vi "test_az_pos.vi"() -> ()   [LabVIEW 2019]
panel:
  out "counts":u64[](graph)
  in  "home":dbl format="%#_13g"
  out "error":dbl[](graph)
  out "graph":dbl[][](graph)
  out "out [deg]":dbl[](array[numeric])
  out "in [deg]":dbl[](array[numeric])
  in  "negate?":bool
  in  "reference":u64=79895940197
  in  "step":u64=4018143232
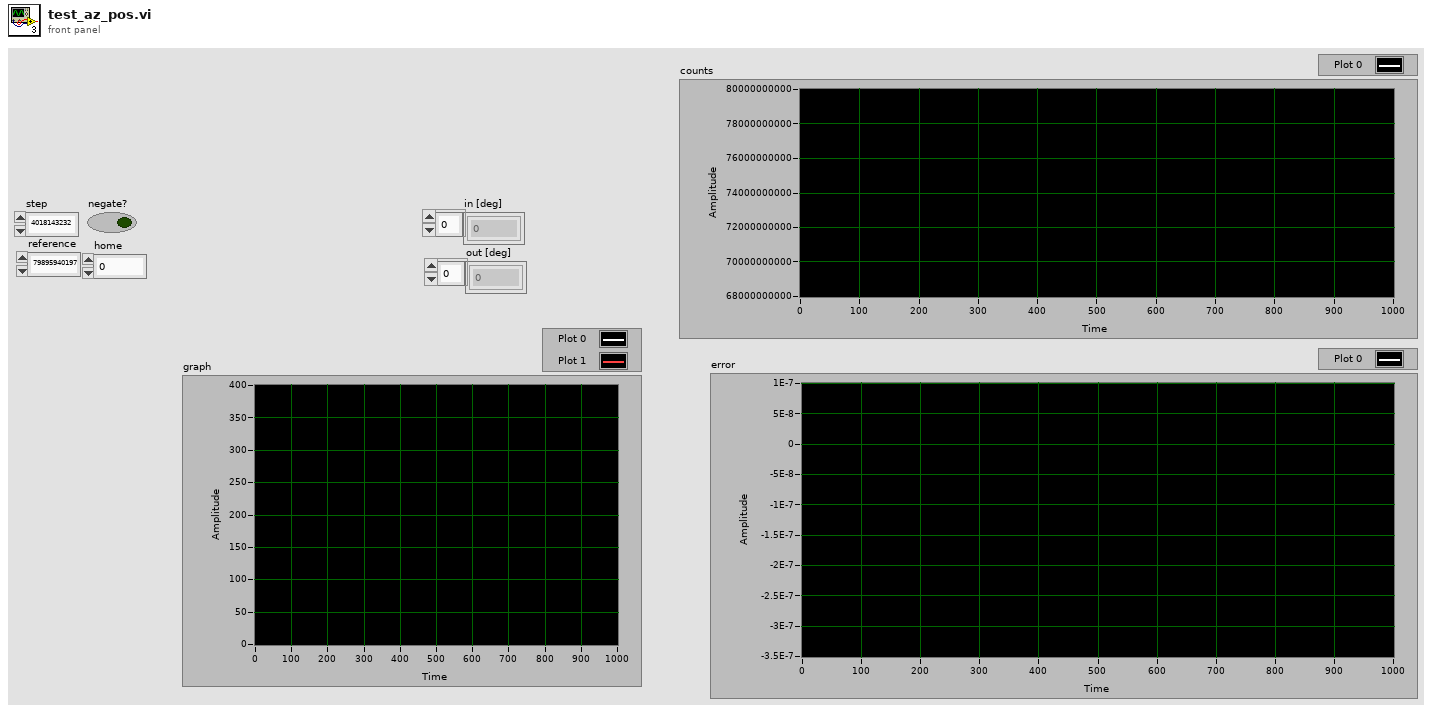
[diagram p1: front panel]
types:
  T1 = cluster{"home":fxp<+/-,32,2>, "counts":u64, "reference":u64, "step":u64, "negate?":bool}
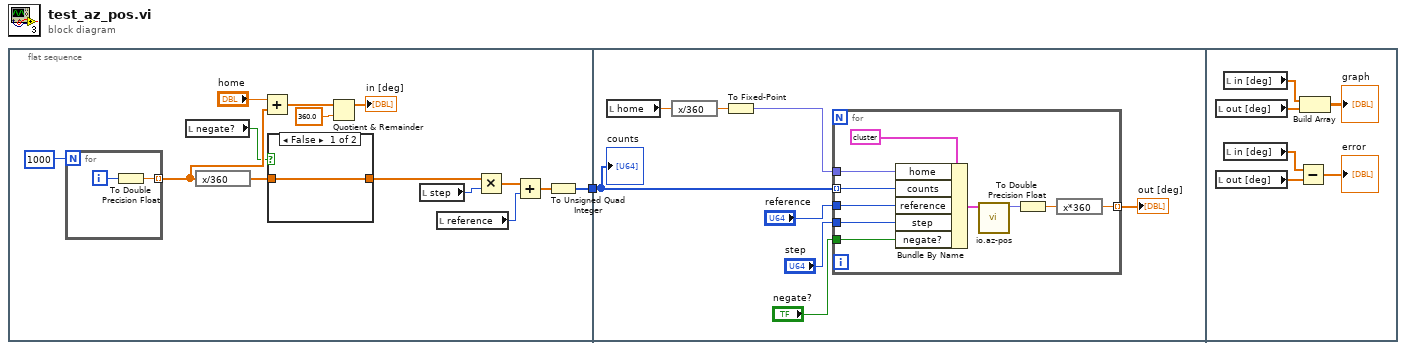
[diagram p0: block diagram]
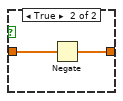
[diagram p2: hidden frame]
diagram:
  n1 = flat-sequence {
    tunnel: [w11] -> w1
    tunnel: w1 -> [w25]
    frame #0 {
      n2 = for {
        N: 1000 -> [_]
        tunnel: [w19] -> w8 mode=indexing
        i -> [w20]
        n3 = To Double Precision Float(number=w20) -> (double precision float=w19:dbl)
      }
      n4 = local read "negate?"() -> (w4:bool)
      n5 = expression code="x/360"(w8) -> (w5:dbl[])
      n6 = Add(x="home", y=w8) -> (x+y=w7:dbl[])
      n7 = case shown="False" w4 {
        tunnel: [w16 w17] -> w3
        tunnel: w5 -> [w16 w18]
        frame False {
        }
        frame True {
          n8 = Negate(x=w18) -> (-x=w17:dbl[])
        }
      }
      n9 = Quotient & Remainder(x=w7, y=360.0) -> (x-y*floor(x/y)=→"in [deg]":dbl[])  [unwired: 1 out]
      n10 = local read "step"() -> (w14:u64)
      n11 = local read "reference"() -> (w13:u64)
      n12 = Multiply(x=w3, y=w14) -> (x*y=w2:dbl[])
      n13 = Add(x=w2, y=w13) -> (x+y=w12:dbl[])
      n14 = To Unsigned Quad Integer(1:w12) -> (0:w11:u64[])
    }
    frame #1 {
      n15 = local read "home"() -> (w23:dbl)
      n16 = expression code="x/360"(w23) -> (w22:dbl)
      n17 = To Fixed-Point(number=w22) -> (fixed-point=w21:fxp<+/-,32,2>)  [unwired: 1 in]
      n18 = for {
        tunnel: [w34] -> w24 mode=indexing
        tunnel: "reference" -> [w33]
        tunnel: "step" -> [w32]
        tunnel: "negate?" -> [w31]
        tunnel: w21 -> [w30]
        tunnel: w25 -> [w29] mode=indexing
        n19 = Bundle By Name(cluster=T1 {"home"=0.0, "counts"=0, "reference"=0, "step"=0, "negate?"=FALSE} ("Cluster"), "home"=w30, "counts"=w29, "reference"=w33, "step"=w32, "negate?"=w31) -> (w37:T1)
        n20 = call "io.az-pos.vi"("Cluster"=w37) -> ("Numeric"=w35:fxp<+/-,32,2>)  [unwired: 10 in]
        n21 = To Double Precision Float(number=w35) -> (double precision float=w36:dbl)
        n22 = expression code="x*360"(w36) -> (w34:dbl)
      }
      "out [deg]" <- w24
      "counts" <- w25
    }
    frame #2 {
      n23 = local read "out [deg]"() -> (w43:dbl[])
      n24 = local read "out [deg]"() -> (w40:dbl[])
      n25 = local read "in [deg]"() -> (w44:dbl[])
      n26 = local read "in [deg]"() -> (w41:dbl[])
      n27 = Subtract(x=w41, y=w40) -> (x-y=→"error":dbl[])
      n28 = Build Array(w44, w43) -> (→"graph":dbl[][])
    }
  }
